vi "VISA_niScope_Fgen_Digital.vi"() -> ()   [LabVIEW 2021]
uses:
  <instrlib>/niScope/Acquire/niScope Multi Read Cluster.vi
  <instrlib>/niDigital/niDigital.llb/niDigital Get Channel Name.vi
  <instrlib>/Tektronix MSO5X Series/Tektronix MSO5X Series.lvlib
panel:
  in  "niDigital_lbl":refnum<k15>="Digital1" caption="niDigital_cap"
  out "channel name":string
  in  "index":i32 min=1
  in  "duration":dbl
  out "Actual Duration":dbl
  in  "I2C Generator Fgen":refnum<k15>
  in  "amplitude":dbl=6.0
  in  "frequency":dbl=6.0
  in  "waveform":T1(ring)=enum."Noise"
  in  "I2C Generator Fgen Channel":string
  in  "Channel(s)":string="0"
  in  "niScope":refnum<k15>="Dev1" caption="Resource Name(s)"
  out "Waveform Graph":T2(graph)
  in  "Simulate?":bool
  in  "Tektronix Scope":refnum<visa-resource-name>
  out "Interpolation Ratio":dbl
  out "Timebase Duration (s)":dbl
  out "Division Number":i32
  in  "Control Type":i32(ring) items=["Horizontal Scale", "Record Length"]
  in  "Sample Rate":dbl=3125000000.0
  in  "Maximum Record Length":dbl=250000000.0 format="%#_6e"
  out "error out":errorcluster
  in  "error in":errorcluster
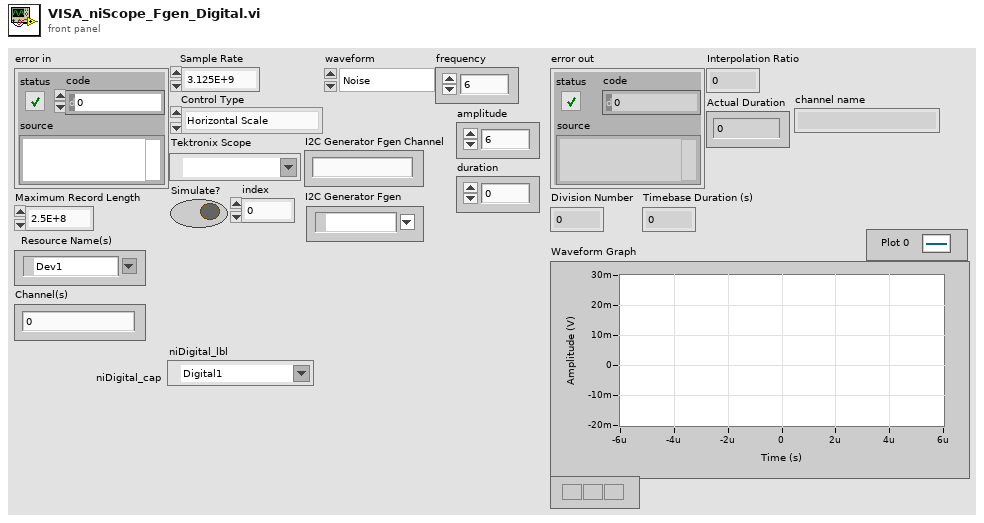
[diagram p1: front panel]
types:
  T1 = enum32{"Sine", "Square", "Triangle", "Ramp Up", "Ramp Down", "DC", "Noise", "User"}
  T2 = cluster{"relativeInitialX":dbl, "xIncrement":dbl, "wfm":dbl[]}[]
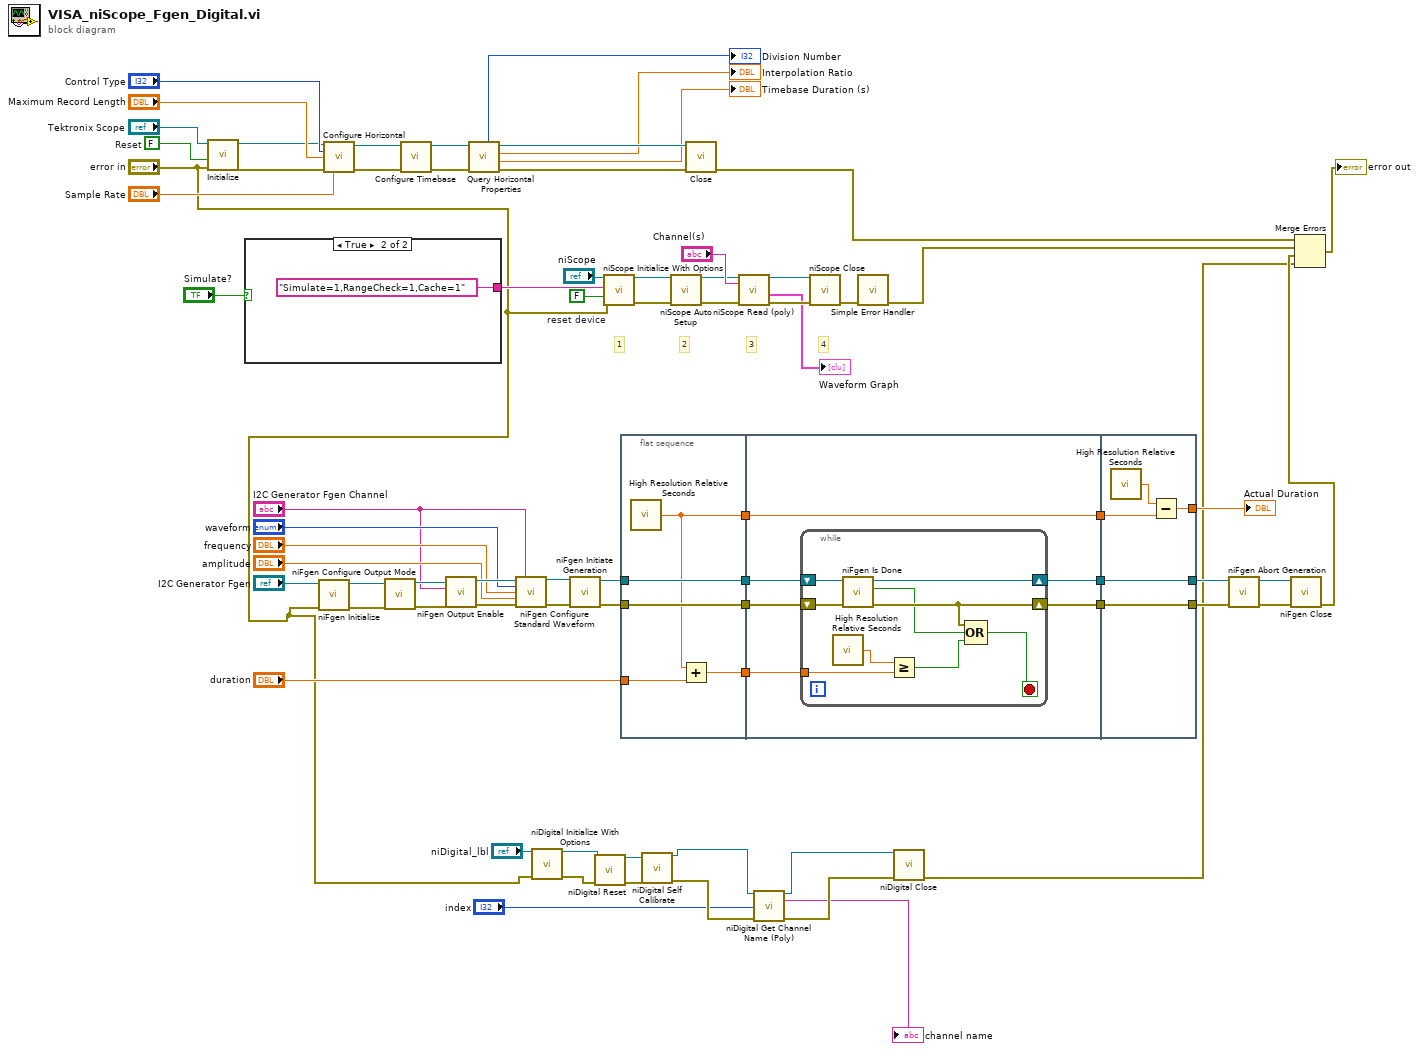
[diagram p0: block diagram]
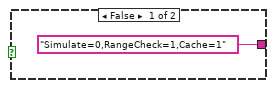
[diagram p2: hidden frame]
diagram:
  w48 = FALSE  # reset device
  w59 = FALSE  # Reset
  # "4"
  # "3"
  # "2"
  # "1"
  n1 = call <instrlib>:"Initialize.vi"("error in (no error)"="error in", "Reset (True)"=w59, "VISA resource name"="Tektronix Scope") -> ("error out"=w61:errorcluster, "VISA resource name out"=w60:refnum<visa-resource-name>)  [unwired: 7 in]
  n2 = case shown="True" "Simulate?" {
    tunnel: ["Simulate=0,RangeCheck=1,Cache=1" ("option string") "Simulate=1,RangeCheck=1,Cache=1" ("option string")] -> w57
    frame False {
    }
    frame True {
    }
  }
  n3 = call <instrlib>:"niFgen Initialize.vi"("error in (no error)"="error in", "Resource Name"="I2C Generator Fgen") -> ("error out"=w32:errorcluster, "Instrument Handle Out"=w35:refnum<k15>)  [unwired: 8 in]
  n4 = call <instrlib>:"Configure Horizontal.vi"("VISA resource name"=w60, "Control Type (0: Horizontal Scale)"="Control Type", "Maximum Record Length (2.5E+8)"="Maximum Record Length", "error in (no error)"=w61, "Sample Rate (3.125E+9)"="Sample Rate") -> ("VISA resource name out"=w70:refnum<visa-resource-name>, "error out"=w71:errorcluster)  [unwired: 9 in]
  n5 = call <instrlib>:"niFgen Configure Output Mode.vi"("error in (no error)"=w32, "Instrument Handle"=w35) -> ("error out"=w22:errorcluster, "Instrument Handle Out"=w31:refnum<k15>)  [unwired: 7 in]
  n6 = call <instrlib>:"Configure Timebase.vi"("error in (no error)"=w71, "VISA resource name"=w70) -> ("error out"=w72:errorcluster, "VISA resource name out"=w73:refnum<visa-resource-name>)  [unwired: 8 in]
  n7 = call <instrlib>:"niFgen Output Enable.vi"("error in (no error)"=w22, "Channel Name"="I2C Generator Fgen Channel", "Instrument Handle"=w31) -> ("error out"=w33:errorcluster, "Instrument Handle Out"=w30:refnum<k15>)  [unwired: 7 in]
  n8 = call <instrlib>:"Query Horizontal Properties.vi"("error in (no error)"=w72, "VISA resource name"=w73) -> ("error out"=w69:errorcluster, "Timebase Duration (s)"=→"Timebase Duration (s)":dbl, "Interpolation Ratio"=→"Interpolation Ratio":dbl, "VISA resource name out"=w68:refnum<visa-resource-name>, "Division Number"=→"Division Number":i32)  [unwired: 5 in]
  n9 = call <instrlib>:"niFgen Configure Standard Waveform.vi"("Instrument Handle"=w30, "Channel Name"="I2C Generator Fgen Channel", "Waveform"="waveform", "Frequency"="frequency", "Amplitude"="amplitude", "error in (no error)"=w33) -> ("Instrument Handle Out"=w29:refnum<k15>, "error out"=w34:errorcluster)  [unwired: 8 in]
  n10 = call <instrlib>:"niDigital Initialize With Options.vi"("resource name"="niDigital_lbl", "error in"="error in") -> ("instrument handle"=w11:refnum<k15>, "error out"=w5:errorcluster)  [unwired: 12 in]
  n11 = call <instrlib>:"niFgen Initiate Generation.vi"("error in (no error)"=w34, "Instrument Handle"=w29) -> ("error out"=w26:errorcluster, "Instrument Handle Out"=w28:refnum<k15>)  [unwired: 8 in]
  n12 = call <instrlib>:"niDigital Reset.vi"("instrument handle in"=w11, "error in"=w5) -> ("instrument handle out"=w13:refnum<k15>, "error out"=w12:errorcluster)  [unwired: 12 in]
  n13 = call <instrlib>:"niScope Initialize With Options.vi"("resource name"="niScope", "option string"=w57, "reset device"=w48, "error in"="error in") -> ("instrument handle"=w45:refnum<k15>, "error out"=w46:errorcluster)  [unwired: 10 in]
  n14 = flat-sequence {
    tunnel: w26 -> [w80]
    tunnel: w28 -> [w81]
    tunnel: [w81] -> w42
    tunnel: [w80] -> w41
    tunnel: [w79] -> w40
    tunnel: "duration" -> [w78]
    tunnel: [w77] -> w39
    tunnel: w42 -> [w87]
    tunnel: w41 -> [w85]
    tunnel: [w86] -> w38
    tunnel: [w84] -> w37
    tunnel: [w83] -> w36
    tunnel: w40 -> [w83]
    tunnel: w39 -> [w82]
    tunnel: [w100] -> w25
    tunnel: [w101] -> w27
    tunnel: w38 -> [w101]
    tunnel: w37 -> [w100]
    tunnel: w36 -> [w98]
    tunnel: [w97] -> w16
    frame #0 {
      n15 = call <vilib>:"High Resolution Relative Seconds.vi"() -> ("relative seconds"=w79:dbl)
      n16 = Add(x=w79, y=w78) -> (x+y=w77:dbl)
    }
    frame #1 {
      n17 = while {
        shift-right: [w95] -> w86
        shift-left: w87 -> [w96]
        shift-right: [w93] -> w84
        shift-left: w85 -> [w94]
        tunnel: w82 -> [w90]
        stop <- w92 stop-if-true
        n18 = call <vilib>:"High Resolution Relative Seconds.vi"() -> ("relative seconds"=w91:dbl)
        n19 = call <instrlib>:"niFgen Is Done.vi"("error in (no error)"=w94, "Instrument Handle"=w96) -> ("error out"=w93:errorcluster, "Done"=w88:bool, "Instrument Handle Out"=w95:refnum<k15>)  [unwired: 7 in]
        n20 = Greater Or Equal?(x=w91, y=w90) -> (x >= y?=w89:bool)
        n21 = Compound Arithmetic op=OR(w93, w88, w89) -> (w92:bool)
      }
    }
    frame #2 {
      n22 = call <vilib>:"High Resolution Relative Seconds.vi"() -> ("relative seconds"=w99:dbl)
      n23 = Subtract(x=w99, y=w98) -> (x-y=w97:dbl)
    }
  }
  n24 = call <instrlib>:"niDigital Self Calibrate.vi"("instrument handle in"=w13, "error in"=w12) -> ("instrument handle out"=w8:refnum<k15>, "error out"=w10:errorcluster)  [unwired: 12 in]
  n25 = call <instrlib>:"niScope Auto Setup.vi"("instrument handle"=w45, "error in"=w46) -> ("instrument handle out"=w49:refnum<k15>, "error out"=w50:errorcluster)  [unwired: 12 in]
  n26 = call <instrlib>:"Close.vi"("error in (no error)"=w69, "VISA resource name"=w68) -> ("error out"=w74:errorcluster)  [unwired: 9 in]
  n27 = call-poly <instrlib>:"niScope Read (poly).vi"("error in"=w50, "channels"="Channel(s)", "instrument handle"=w49) -> ("error out"=w53:errorcluster, "waveform"=→"Waveform Graph":T2, "instrument handle out"=w54:refnum<k15>)  [unwired: 5 in, 1 out]
  n28 = call-poly <instrlib>:"niDigital Get Channel Name (Poly).vi"("instrument handle in"=w8, "index"="index", "error in"=w10) -> ("instrument handle out"=w9:refnum<k15>, "channel name"=→"channel name":string, "error out"=w7:errorcluster)  [unwired: 10 in]
  n29 = call <instrlib>:"niScope Close.vi"("instrument handle"=w54, "error in"=w53) -> ("error out"=w55:errorcluster)  [unwired: 13 in]
  n30 = call <vilib>:"Simple Error Handler.vi"("error in (no error)"=w55) -> ("error out"=w43:errorcluster)  [unwired: 4 in, 4 out]
  n31 = call <instrlib>:"niDigital Close.vi"("instrument handle"=w9, "error in"=w7) -> ("error out"=w2:errorcluster)  [unwired: 13 in]
  n32 = call <instrlib>:"niFgen Abort Generation.vi"("error in (no error)"=w25, "Instrument Handle"=w27) -> ("error out"=w23:errorcluster, "Instrument Handle Out"=w24:refnum<k15>)  [unwired: 8 in]
  n33 = call <instrlib>:"niFgen Close.vi"("error in (no error)"=w23, "Instrument Handle"=w24) -> ("error out"=w14:errorcluster)  [unwired: 9 in]
  n34 = Merge Errors(w74, w43, w14, w2) -> (→"error out":errorcluster)
  "Actual Duration" <- w16
